vi "toFahrenheit.vi"(11 "degC":dbl) -> (3 "degF":dbl)   [LabVIEW 2014]
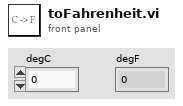
[diagram p1: front panel]
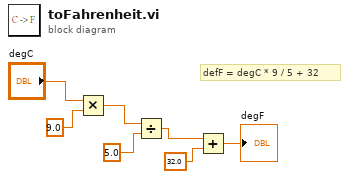
[diagram p0: block diagram]
diagram:
  # "defF = degC * 9 / 5 + 32"
  n1 = Multiply(x="degC", y=9.0) -> (x*y=w5:dbl)
  n2 = Divide(x=w5, y=5.0) -> (x/y=w6:dbl)
  n3 = Add(x=w6, y=32.0) -> (x+y=→"degF":dbl)
